vi "Actor Core.vi"(8 "error in":errorcluster, 11 "Nested in":refnum<class "UI Actor.lvclass">) -> (0 "error out":errorcluster, 3 "Actor out":refnum<class "Actor.lvclass">)   [LabVIEW 2020, in "UI Actor.lvlib" / "UI Actor.lvclass"]
doc: "(<B>Filename</B>: Actor Framework.lvlib:Actor.lvclass:Actor Core.vi)\n\nReceives messages to the actor, reacts to them, and initiates any error handling that may shut the actor down.\n\nDescendant classes may override this VI to append parallel tasks for the actor to complete while it handles messages. Overrides use the Call Parent Method node."
uses:
  UI Actor.lvclass
  C:/Program Files (x86)/National Instruments/LabVIEW 2020/vi.lib/ActorFramework/Actor/Actor.lvclass
  <vilib>/ActorFramework/Actor/Actor.lvclass
  Message Actor/Message Actor.lvclass
  C:/Users/eddiews/Documents/Git Hub Repositorios/VendingMachine_ActorFramework/SubPanel Actor/SubPanel Actor/SubPanel Actor.lvclass
  Coins Actor/Coins Actor.lvclass
  <vilib>/ActorFramework/Actor/Actor.lvclass/Actor.ctl
  <vilib>/ActorFramework/Message Enqueuer/Message Enqueuer.lvclass/Message Enqueuer.ctl
  UI Actor.lvclass/UI Actor.ctl
  SubPanel Actor/SubPanel Actor/SubPanel Actor.lvclass/SubPanel Actor.ctl
  <vilib>/ActorFramework/Message Enqueuer/Init from Existing Queue.vi
  <vilib>/ActorFramework/Message Enqueuer/Enqueue.vi
  SubPanel Actor/SubPanel Actor/SubPanel Actor.lvclass
  <vilib>/ActorFramework/Stop Msg/Stop Msg.lvclass
  C:/Program Files (x86)/National Instruments/LabVIEW 2020/vi.lib/ActorFramework/Message/Message.lvclass
  <vilib>/ActorFramework/Message Priority Queue/Priority Enqueue.vi
  <vilib>/ActorFramework/Message Enqueuer/Message Enqueuer.lvclass
  C:/Users/eddiews/Documents/Git Hub Repositorios/VendingMachine_ActorFramework/UI Actor/UI Actor.lvclass
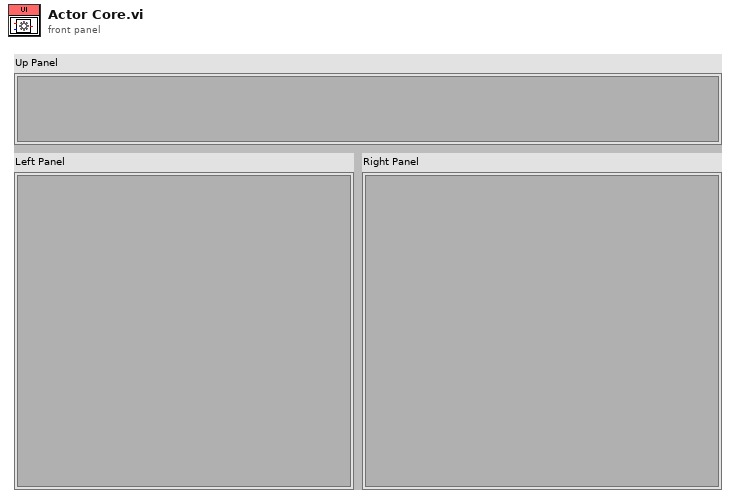
[diagram p1: front panel]
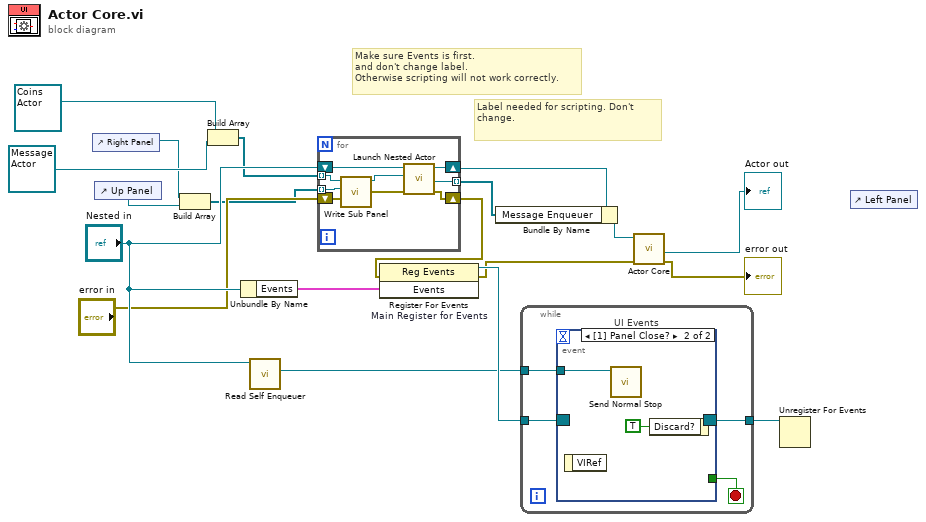
[diagram p0: block diagram]
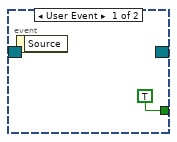
[diagram p2: hidden frame]
diagram:
  # "Label needed for scripting. Don't change."
  # "Make sure Events is first.\nand don't change label.\nOtherwise scripting will not work correctly."
  n1 = control-ref of="Right Panel"() -> (w6:refnum<vi>)
  n2 = control-ref of="Up Panel"() -> (w5:refnum<vi>)
  n3 = Build Array(w6, w5) -> (w4:refnum<vi>[])
  n4 = Build Array(refnum<class "Coins Actor.lvclass"> refnum ("Coins Actor.lvlib:Coins Actor.lvclass"), refnum<class "Message Actor.lvclass"> refnum ("Message Actor.lvlib:Message Actor.lvclass")) -> (w7:refnum<class "SubPanel Actor.lvclass">[])
  n5 = Unbundle By Name("Nested in") -> ("Events"=w16:cluster{"Stop":refnum<user-event>})
  n6 = call <vilib>:"Read Self Enqueuer.vi"("Actor"="Nested in") -> ("Self Enqueuer"=w14:refnum<class "Message Enqueuer.lvclass">)  [unwired: 10 in]
  n7 = for {
    tunnel: w7 -> [w22] mode=indexing
    tunnel: w4 -> [w23] mode=indexing
    shift-right: [w27] -> w10
    shift-left: "error in" -> [w26]
    shift-right: [w28] -> w3
    shift-left: "Nested in" -> [w24]
    tunnel: [w20] -> w2 mode=indexing
    n8 = call "Write Sub Panel.vi"("error in (no error)"=w26, "Sub Panel"=w23, "SubPanel Actor in"=w22) -> ("error out"=w25:errorcluster, "SubPanel Actor out"=w21:refnum<class "SubPanel Actor.lvclass">)  [unwired: 7 in]
    n9 = call <vilib>:"Launch Nested Actor.vi"("error in (no error)"=w25, "Nested Actor"=w21, "Caller Actor in"=w24) -> ("error out"=w27:errorcluster, "Nested Actor's Enqueuer"=w20:refnum<class "Message Enqueuer.lvclass">, "Caller Actor out"=w28:refnum<class "UI Actor.lvclass">)  [unwired: 6 in]
  }
  n10 = register-events "Main Register for Events"(error in=w10, w16) -> (reference out=w17:refnum<event-registration>, error out=w13:errorcluster)  [unwired: 1 in]
  n11 = Bundle By Name(cluster=w3, "Message Enqueuer"=w2) -> (w1:refnum<class "UI Actor.lvclass">)
  n12 = while {
    tunnel: w17 -> [w32]
    tunnel: [w30] -> w15
    tunnel: w14 -> [w29]
    stop <- w31 stop-if-true
    n13 = event "UI Events" shown="[1] Panel Close?" {
      selector: w32 -> [_ _]
      dyn-events: [_ _] -> w30
      timeout: _ -> [_ _]
      tunnel: [TRUE _] -> w31
      tunnel: w29 -> [_ w34]
      event User Event {
        n14 = event-data() -> ()  [unwired: 1 in, 1 out]
      }
      event Panel Close? {
        n15 = event-data() -> ()  [unwired: 1 in, 1 out]
        n16 = call <vilib>:"Send Normal Stop.vi"("Message Enqueuer"=w34) -> ()  [unwired: 10 in, 1 out]
        n17 = event-data("Discard?"=TRUE) -> ()  [unwired: 1 in, 1 out]
      }
    }
  }
  n18 = call-parent "Actor Core.vi"("error in"=w13, "Actor in"=w1) -> ("error out"=→"error out":errorcluster, "Actor out"=→"Actor out":refnum<class "Actor.lvclass">)  [unwired: 8 in]
  n19 = Unregister For Events(event registration refnum=w15) -> ()  [unwired: 1 in, 1 out]
  n20 = control-ref of="Left Panel"() -> ()  [unwired: 1 out]
